vi "Is Current ROI Tool Zoom, Pan or Ellipse.vi"(8 "Error In":errorcluster, 11 "Current ROI Tool":T2 items=["Zoom Tool"=8, "Selection Tool"=0, "Pan Tool"=9, "Point Tool"=1, "Line Tool"=2, "Rectangle Tool"=3, "Rotated Rectangle Tool"=12, "Polyline Tool"=10, "Polygon Tool"=5, "Freehand Tool"=11, "Closed Freehand Tool"=6, "Ellipse Tool"=4, "Annulus Tool"=7]) -> (0 "Error Out":errorcluster, 3 "Processed ROI Types":T1)   [LabVIEW 2021, in "Image.lvlib"]
uses:
  Image.lvlib
  Image Selection Tool.ctl
  Processed ROI Types.ctl
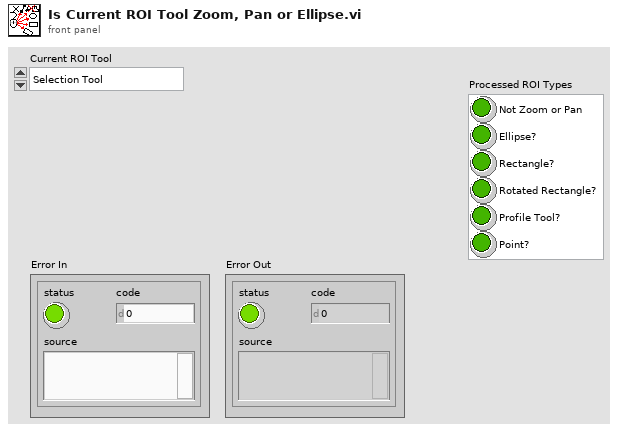
[diagram p1: front panel]
types:
  T1 = typedef "Image.lvlib/Processed ROI Types.ctl" = cluster{"Not Zoom or Pan":bool, "Ellipse?":bool, "Rectangle?":bool, "Rotated Rectangle?":bool, "Profile Tool?":bool, "Point?":bool}
  T2 = typedef "Image.lvlib/Image Selection Tool.ctl" = u32
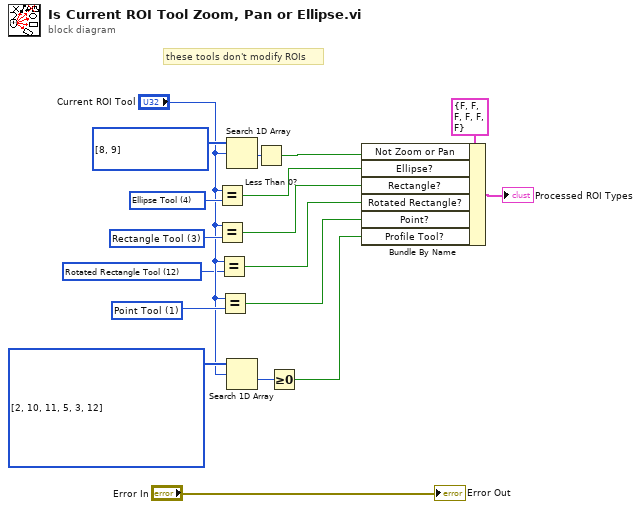
[diagram p0: block diagram]
diagram:
  w9 = T2 12 items=["Zoom Tool"=8, "Selection Tool"=0, "Pan Tool"=9, "Point Tool"=1, "Line Tool"=2, "Rectangle Tool"=3, "Rotated Rectangle Tool"=12, "Polyline Tool"=10, "Polygon Tool"=5, "Freehand Tool"=11, "Closed Freehand Tool"=6, "Ellipse Tool"=4, "Annulus Tool"=7] ("Current ROI Tool")
  w12 = T2[] [2, 10, 11, 5, 3, 12] items=["Zoom Tool"=8, "Selection Tool"=0, "Pan Tool"=9, "Point Tool"=1, "Line Tool"=2, "Rectangle Tool"=3, "Rotated Rectangle Tool"=12, "Polyline Tool"=10, "Polygon Tool"=5, "Freehand Tool"=11, "Closed Freehand Tool"=6, "Ellipse Tool"=4, "Annulus Tool"=7] ("Current ROI Tool")
  w13 = T2 1 items=["Zoom Tool"=8, "Selection Tool"=0, "Pan Tool"=9, "Point Tool"=1, "Line Tool"=2, "Rectangle Tool"=3, "Rotated Rectangle Tool"=12, "Polyline Tool"=10, "Polygon Tool"=5, "Freehand Tool"=11, "Closed Freehand Tool"=6, "Ellipse Tool"=4, "Annulus Tool"=7] ("Current ROI Tool")
  w14 = T2 3 items=["Zoom Tool"=8, "Selection Tool"=0, "Pan Tool"=9, "Point Tool"=1, "Line Tool"=2, "Rectangle Tool"=3, "Rotated Rectangle Tool"=12, "Polyline Tool"=10, "Polygon Tool"=5, "Freehand Tool"=11, "Closed Freehand Tool"=6, "Ellipse Tool"=4, "Annulus Tool"=7] ("Current ROI Tool")
  w15 = T2 4 items=["Zoom Tool"=8, "Selection Tool"=0, "Pan Tool"=9, "Point Tool"=1, "Line Tool"=2, "Rectangle Tool"=3, "Rotated Rectangle Tool"=12, "Polyline Tool"=10, "Polygon Tool"=5, "Freehand Tool"=11, "Closed Freehand Tool"=6, "Ellipse Tool"=4, "Annulus Tool"=7] ("Current ROI Tool")
  w17 = T2[] [8, 9] items=["Zoom Tool"=8, "Selection Tool"=0, "Pan Tool"=9, "Point Tool"=1, "Line Tool"=2, "Rectangle Tool"=3, "Rotated Rectangle Tool"=12, "Polyline Tool"=10, "Polygon Tool"=5, "Freehand Tool"=11, "Closed Freehand Tool"=6, "Ellipse Tool"=4, "Annulus Tool"=7] ("Current ROI Tool")
  # "these tools don't modify ROIs"
  n1 = Equal?(x="Current ROI Tool", y=w15) -> (x = y?=w6:bool)
  n2 = Equal?(x="Current ROI Tool", y=w14) -> (x = y?=w5:bool)
  n3 = Equal?(x="Current ROI Tool", y=w9) -> (x = y?=w4:bool)
  n4 = Equal?(x="Current ROI Tool", y=w13) -> (x = y?=w3:bool)
  n5 = Search 1D Array(1D array=w17, element="Current ROI Tool") -> (index of element=w18:i32)  [unwired: 1 in]
  n6 = Search 1D Array(1D array=w12, element="Current ROI Tool") -> (index of element=w11:i32)  [unwired: 1 in]
  n7 = Less Than 0?(x=w18) -> (x < 0?=w7:bool)
  n8 = Greater Or Equal To 0?(x=w11) -> (x >= 0?=w2:bool)
  n9 = Bundle By Name(cluster=T1 {"Not Zoom or Pan"=FALSE, "Ellipse?"=FALSE, "Rectangle?"=FALSE, "Rotated Rectangle?"=FALSE, "Profile Tool?"=FALSE, "Point?"=FALSE} ("ROI Types"), "Not Zoom or Pan"=w7, "Ellipse?"=w6, "Rectangle?"=w5, "Rotated Rectangle?"=w4, "Point?"=w3, "Profile Tool?"=w2) -> (→"Processed ROI Types":T1)
  "Error Out" <- "Error In"
